vi "Register For Events.vi"(8 "error in (no error)":errorcluster, 10 "Events To Register":T3[](array[typedef]), 11 "Session in":refnum<class "Plugin Session.lvclass">) -> (0 "error out":errorcluster, 1 "Plugin Events":T1, 2 "Event Refnum":T2, 3 "Session out":refnum<class "Plugin Session.lvclass">)   [LabVIEW 2021, in "InstrumentStudio Plugin SDK.lvlib" / "Plugin Session.lvclass"]
doc: "Call this VI to let the framework know which events you want to get notifications for. Only pass in events that you are going to handle in your event structure. There are four events available:\n\nShutdown\nThis event is fired when the document containing this VI is closing. The plugin must close all references and stop the VI. If the VI does not stop within a few seconds, the document will prompt the user to abort the running VI.\n\nProject Saved\nThis event is fired when the path of the Project changes. It passes event data for the updated project path and a Completion Id. The plugin must call Notify Event Complete with this Completion Id to let the framework know its processing is complete. Failure to do this will result in a hang.\n\nStop All Outputs\nThe Stop All Outputs event is fired when the 'Stop all outputs' button is pressed on the document toolbar. It notifies the plugin that it should cease sending output data to any external devices.\n\nGeneric Message\nReserved for internal/future use by InstrumentStudio."
uses:
  Plugin Session.lvclass
  Plugin Events Enum.ctl
  Event Registration Refnum.ctl
  Plugin Events.ctl
  Plugin Session.lvclass/Plugin Session.ctl
  Read Session Id.vi
  Read Plugin Events.vi
  Read Event Refnum.vi
  NationalInstruments.VIHost.Interop.dll
  InstrumentStudio Plugin SDK.lvlib
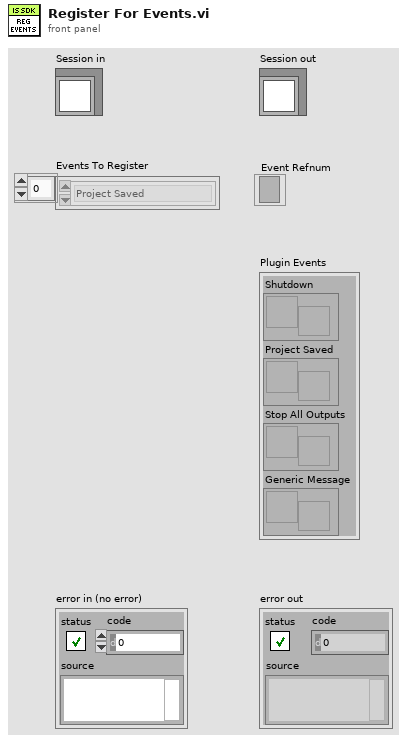
[diagram p1: front panel]
types:
  T1 = typedef "InstrumentStudio Plugin SDK.lvlib/Plugin Events.ctl" = cluster{"Shutdown":refnum<user-event>, "Project Saved":refnum<user-event>, "Stop All Outputs":refnum<user-event>, "Generic Message":refnum<user-event>}
  T2 = typedef "InstrumentStudio Plugin SDK.lvlib/Event Registration Refnum.ctl" = refnum<event-registration>
  T3 = typedef "InstrumentStudio Plugin SDK.lvlib/Plugin Events Enum.ctl" = enum16{"Shutdown", "Project Saved", "Stop All Outputs", "Generic Message"}
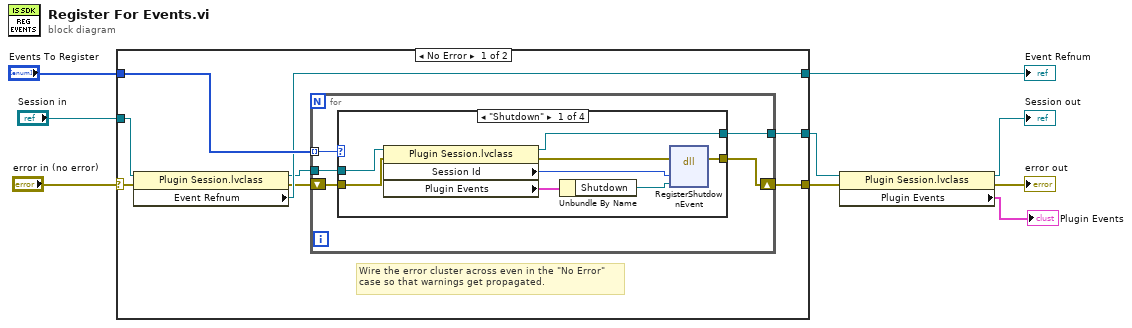
[diagram p0: block diagram]
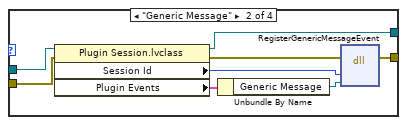
[diagram p2: hidden frame]
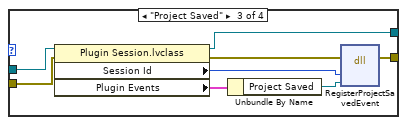
[diagram p3: hidden frame]
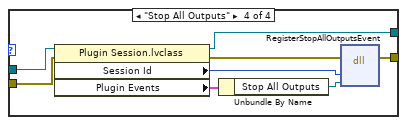
[diagram p4: hidden frame]
diagram:
  n1 = case shown="No Error" "error in (no error)" {
    selector: "error in (no error)" -> [w12 w56]
    tunnel: [w16 w56] -> w8
    tunnel: [w10 w55] -> w3
    tunnel: "Session in" -> [w14 w55]
    tunnel: "Events To Register" -> [w17 _]
    tunnel: [w15 _] -> w5
    frame No Error {
      # "Wire the error cluster across even in the \"No Error\"\ncase so that warnings get propagated."
      n2 = property class="Plugin Session.lvclass"(reference=w14, error in=w12) -> (reference out=w13:refnum<class "Plugin Session.lvclass">, error out=w11:errorcluster, "Event Refnum"=w15:T2)
      n3 = for {
        tunnel: w17 -> [w22] mode=indexing
        tunnel: w13 -> [w21]
        shift-right: [w19] -> w16
        shift-left: w11 -> [w20]
        tunnel: [w18] -> w10
        n4 = case shown="\"Shutdown\"" w22 {
          tunnel: w21 -> [w25 w34 w43 w50]
          tunnel: w20 -> [w26 w33 w42 w49]
          tunnel: [w23 w31 w40 w48] -> w19
          tunnel: [w24 w32 w39 w47] -> w18
          frame "Shutdown" {
            n5 = property class="Plugin Session.lvclass"(reference=w25, error in=w26) -> (reference out=w24:refnum<class "Plugin Session.lvclass">, error out=w30:errorcluster, "Session Id"=w27:u64, "Plugin Events"=w28:T1)
            n6 = Unbundle By Name(w28) -> ("Shutdown"=w29:refnum<user-event>)
            n7 = dll-call lib="C:/git/srd-adg-rf/dst/dstd/DSTInstStudio/source/utilities/PluginSDK/NationalInstruments.VIHost.Interop.dll" fn="RegisterShutdownEvent"(error in=w30, "hostId"=w27, "eventRef"=w29) -> (error out=w23:errorcluster)  [unwired: 5 in, 1 out]
          }
          frame "Generic Message" {
            n8 = property class="Plugin Session.lvclass"(reference=w34, error in=w33) -> (reference out=w32:refnum<class "Plugin Session.lvclass">, error out=w38:errorcluster, "Session Id"=w35:u64, "Plugin Events"=w36:T1)
            n9 = Unbundle By Name(w36) -> ("Generic Message"=w37:refnum<user-event>)
            n10 = dll-call lib="C:/git/srd-adg-rf/dst/dstd/DSTInstStudio/source/utilities/PluginSDK/NationalInstruments.VIHost.Interop.dll" fn="RegisterGenericMessageEvent"(error in=w38, "hostId"=w35, "eventRef"=w37) -> (error out=w31:errorcluster)  [unwired: 5 in, 1 out]
          }
          frame "Project Saved" {
            n11 = property class="Plugin Session.lvclass"(reference=w43, error in=w42) -> (reference out=w39:refnum<class "Plugin Session.lvclass">, error out=w41:errorcluster, "Session Id"=w46:u64, "Plugin Events"=w45:T1)
            n12 = Unbundle By Name(w45) -> ("Project Saved"=w44:refnum<user-event>)
            n13 = dll-call lib="C:/git/srd-adg-rf/dst/dstd/DSTInstStudio/source/utilities/PluginSDK/NationalInstruments.VIHost.Interop.dll" fn="RegisterProjectSavedEvent" ("NationalInstruments.VIHost.Interop.dll:RegisterNamedCommandEvent")(error in=w41, "hostId"=w46, "projectSavedEventRef"=w44) -> (error out=w40:errorcluster)  [unwired: 5 in, 1 out]
          }
          frame "Stop All Outputs" {
            n14 = property class="Plugin Session.lvclass"(reference=w50, error in=w49) -> (reference out=w47:refnum<class "Plugin Session.lvclass">, error out=w51:errorcluster, "Session Id"=w54:u64, "Plugin Events"=w53:T1)
            n15 = Unbundle By Name(w53) -> ("Stop All Outputs"=w52:refnum<user-event>)
            n16 = dll-call lib="C:/git/srd-adg-rf/dst/dstd/DSTInstStudio/source/utilities/PluginSDK/NationalInstruments.VIHost.Interop.dll" fn="RegisterStopAllOutputsEvent"(error in=w51, "hostId"=w54, "eventRef"=w52) -> (error out=w48:errorcluster)  [unwired: 5 in, 1 out]
          }
        }
      }
    }
    frame Error {
    }
  }
  "Event Refnum" <- w5
  n17 = property class="Plugin Session.lvclass"(reference=w3, error in=w8) -> (reference out=→"Session out":refnum<class "Plugin Session.lvclass">, error out=→"error out":errorcluster, "Plugin Events"=→"Plugin Events":T1)
